vi "IMU.vi"(8 "error in (no error)":errorcluster, 10 "Acc/Gyro  address":u8, 11 "I2C Ref":T1) -> (3 "error out":errorcluster, 5 "IMU Acc":cluster{dbl, dbl, dbl}(graph), 6 "IMU Gyro":cluster{dbl, dbl, dbl}(graph))   [LabVIEW 2019]
uses:
  <vilib>/myRIO/Instrument Drivers/Onboard IO/I2C/typedefs/I2C Reference.ctl
  <vilib>/myRIO/Common/Instrument Driver Framework/Utilities/typedefs/myRIO Generic Hardware Reference.ctl
  <vilib>/myRIO/Common/Instrument Driver Framework/Utilities/typedefs/Hardware Version Enum.ctl
  <vilib>/myRIO/Common/Instrument Driver Framework/Utilities/typedefs/myRIO v1.0 Reference.ctl
  <vilib>/myRIO/Common/Instrument Driver Framework/Utilities/typedefs/Generic FPGA Reference.ctl
  <vilib>/myRIO/Common/Instrument Driver Framework/myRIO v1.0/I2C/typedefs/I2C Channels Enum.ctl
  <vilib>/myRIO/Instrument Drivers/Onboard IO/I2C/typedefs/I2C Configuration.ctl
  <vilib>/myRIO/Instrument Drivers/Onboard IO/I2C/typedefs/I2C Transfer Rate.ctl
  <vilib>/Utility/error.llb/Error Cluster From Error Code.vi
  <vilib>/myRIO/Common/Instrument Driver Framework/myRIO v1.0/I2C/vis/myRIO v1.0 Write I2C.vi
  <vilib>/myRIO/Common/Instrument Driver Framework/myRIO v1.0/I2C/vis/myRIO v1.0 Read I2C.vi
  <vilib>/myRIO/Instrument Drivers/Onboard IO/I2C/I2C.lvlib
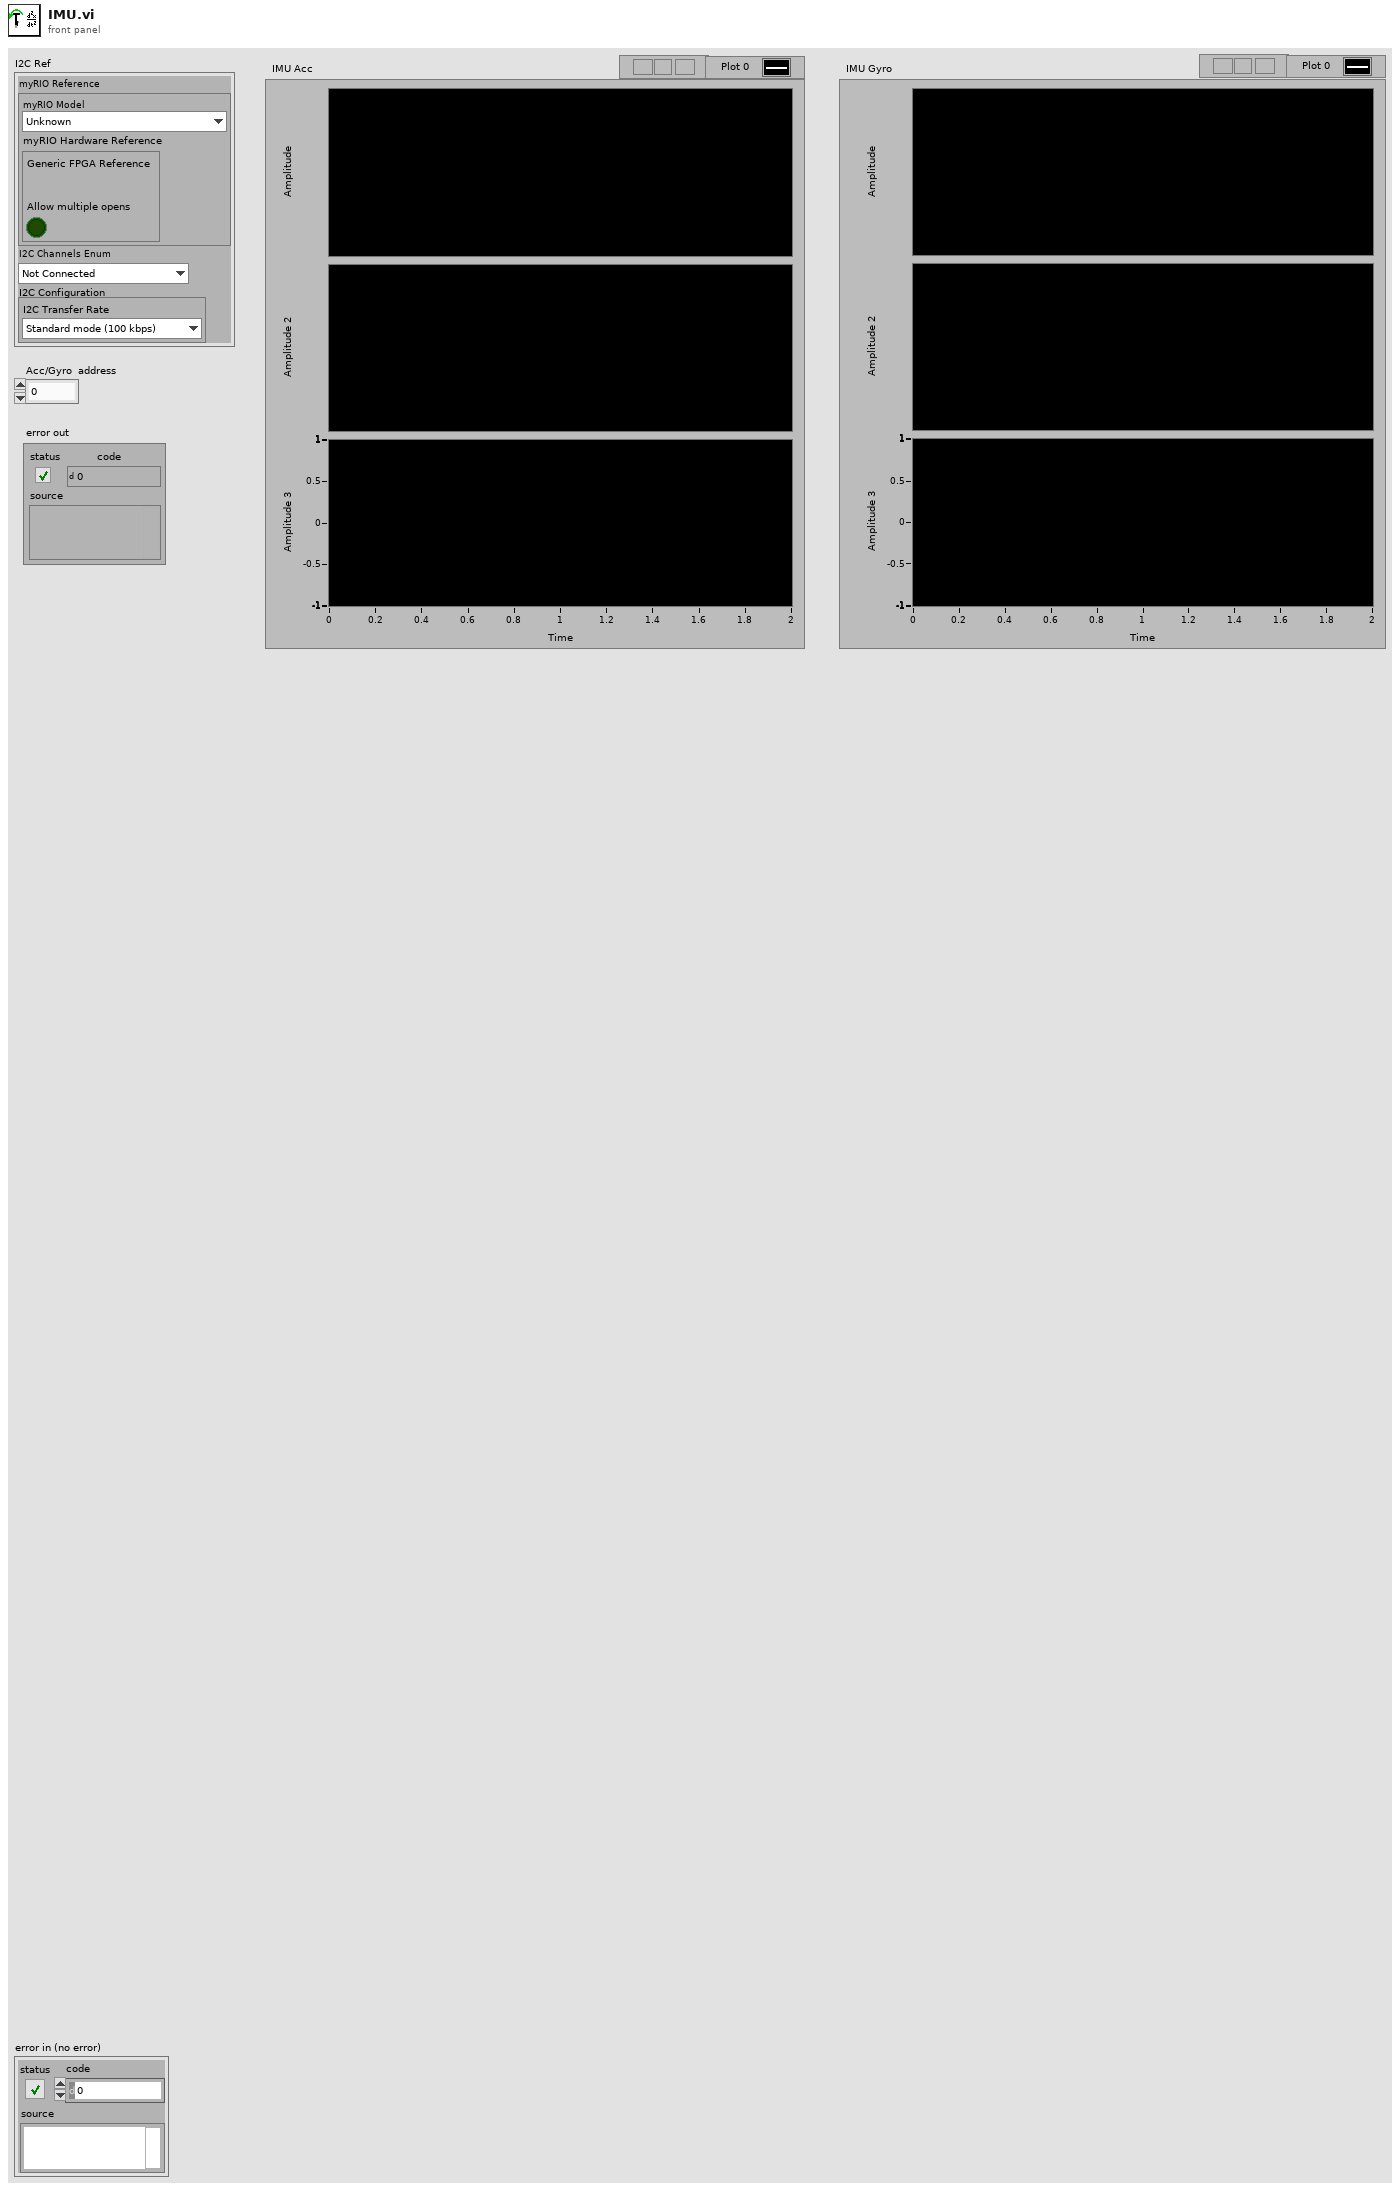
[diagram p1: front panel]
types:
  T1 = typedef "I2C.lvlib/I2C Reference.ctl" = cluster{"myRIO Reference":T2, "I2C Channels Enum":T6, "I2C Configuration":T7}
  T2 = typedef "myRIO Generic Hardware Reference.ctl" = cluster{"myRIO Model":T3, "myRIO Hardware Reference":T4}
  T3 = typedef "Hardware Version Enum.ctl" = enum16{"Unknown", "myRIO-1900", "myRIO-1950", "roboRIO", "NI ELVIS RIO CM", "ELVIS III"}
  T4 = typedef "myRIO v1.0 Reference.ctl" = cluster{"Generic FPGA Reference":T5, "Allow multiple opens":bool}
  T5 = typedef "Generic FPGA Reference.ctl" = refnum<k20>
  T6 = typedef "I2C Channels Enum.ctl" = enum16{"Not Connected", "A/I2C", "B/I2C", "I2C/I2C"}
  T7 = typedef "I2C.lvlib/I2C Configuration.ctl" = cluster{"I2C Transfer Rate":T8}
  T8 = typedef "I2C.lvlib/I2C Transfer Rate.ctl" = enum16{"Standard mode (100 kbps)", "Fast mode (400 kbps)"}
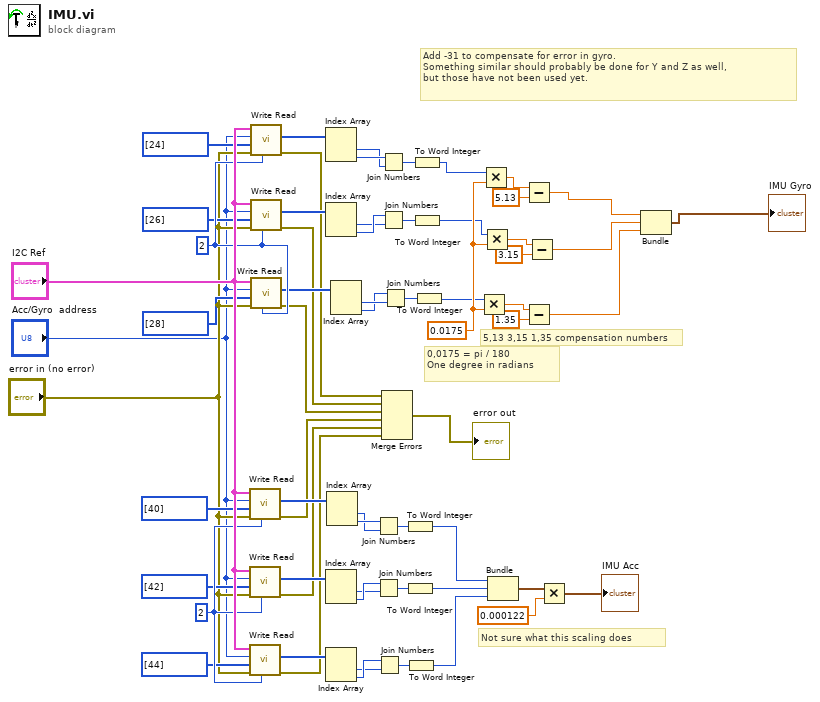
[diagram p0: block diagram]
diagram:
  w13 = 0.0175 ("y")
  w55 = u32 2 ("Byte Count")
  w41 = u32 2 ("Byte Count")
  # "5,13 3,15 1,35 compensation numbers"
  # "Add -31 to compensate for error in gyro.\nSomething similar should probably be done for Y and Z as well,\nbut those have not been used yet."
  # "0,0175 = pi / 180\nOne degree in radians"
  # "Not sure what this scaling does"
  n1 = call <vilib>:"Write Read.vi"("Byte Count"=w41, "error in (no error)"="error in (no error)", "Bytes to Write"=u8[] [40], "Slave Address (7-bit)"="Acc/Gyro  address", "I2C Ref In"="I2C Ref") -> ("error out"=w20:errorcluster, "Bytes Read"=w33:u8[])  [unwired: 3 in, 1 out]
  n2 = call <vilib>:"Write Read.vi"("Byte Count"=w41, "error in (no error)"="error in (no error)", "Bytes to Write"=u8[] [42], "Slave Address (7-bit)"="Acc/Gyro  address", "I2C Ref In"="I2C Ref") -> ("error out"=w19:errorcluster, "Bytes Read"=w31:u8[])  [unwired: 3 in, 1 out]
  n3 = call <vilib>:"Write Read.vi"("Byte Count"=w41, "error in (no error)"="error in (no error)", "Bytes to Write"=u8[] [44], "Slave Address (7-bit)"="Acc/Gyro  address", "I2C Ref In"="I2C Ref") -> ("error out"=w18:errorcluster, "Bytes Read"=w29:u8[])  [unwired: 3 in, 1 out]
  n4 = call <vilib>:"Write Read.vi"("Byte Count"=w55, "error in (no error)"="error in (no error)", "Bytes to Write"=u8[] [24], "Slave Address (7-bit)"="Acc/Gyro  address", "I2C Ref In"="I2C Ref") -> ("error out"=w23:errorcluster, "Bytes Read"=w49:u8[])  [unwired: 3 in, 1 out]
  n5 = call <vilib>:"Write Read.vi"("Byte Count"=w55, "error in (no error)"="error in (no error)", "Bytes to Write"=u8[] [26], "Slave Address (7-bit)"="Acc/Gyro  address", "I2C Ref In"="I2C Ref") -> ("error out"=w22:errorcluster, "Bytes Read"=w47:u8[])  [unwired: 3 in, 1 out]
  n6 = call <vilib>:"Write Read.vi"("Byte Count"=w55, "error in (no error)"="error in (no error)", "Bytes to Write"=u8[] [28], "Slave Address (7-bit)"="Acc/Gyro  address", "I2C Ref In"="I2C Ref") -> ("error out"=w21:errorcluster, "Bytes Read"=w45:u8[])  [unwired: 3 in, 1 out]
  n7 = Index Array "Index Array"(array=w49) -> (element #1=w51:u8, element #2=w52:u8)  [unwired: 2 in]
  n8 = Index Array "Index Array"(array=w47) -> (element #1=w53:u8, element #2=w54:u8)  [unwired: 2 in]
  n9 = Index Array "Index Array"(array=w31) -> (element #1=w37:u8, element #2=w38:u8)  [unwired: 2 in]
  n10 = Index Array "Index Array"(array=w29) -> (element #1=w39:u8, element #2=w40:u8)  [unwired: 2 in]
  n11 = Index Array "Index Array"(array=w33) -> (element #1=w35:u8, element #2=w36:u8)  [unwired: 2 in]
  n12 = Index Array "Index Array"(array=w45) -> (element #1=w16:u8, element #2=w15:u8)  [unwired: 2 in]
  n13 = Join Numbers(hi=w36, lo=w35) -> ((hi.lo)=w26:u16)
  n14 = Join Numbers(hi=w38, lo=w37) -> ((hi.lo)=w27:u16)
  n15 = Join Numbers(hi=w40, lo=w39) -> ((hi.lo)=w28:u16)
  n16 = Join Numbers(hi=w52, lo=w51) -> ((hi.lo)=w42:u16)
  n17 = Join Numbers(hi=w54, lo=w53) -> ((hi.lo)=w43:u16)
  n18 = Join Numbers(hi=w15, lo=w16) -> ((hi.lo)=w44:u16)
  n19 = Merge Errors(w23, w22, w21, w20, w19, w18) -> (→"error out":errorcluster)
  n20 = To Word Integer(number=w26) -> (16bit integer=w61:i16)
  n21 = To Word Integer(number=w27) -> (16bit integer=w60:i16)
  n22 = To Word Integer(number=w28) -> (16bit integer=w59:i16)
  n23 = To Word Integer(number=w42) -> (16bit integer=w14:i16)
  n24 = To Word Integer(number=w43) -> (16bit integer=w12:i16)
  n25 = To Word Integer(number=w44) -> (16bit integer=w11:i16)
  n26 = Multiply(x=w11, y=w13) -> (x*y=w5:dbl)
  n27 = Multiply(x=w14, y=w13) -> (x*y=w10:dbl)
  n28 = Multiply(x=w12, y=w13) -> (x*y=w4:dbl)
  n29 = Bundle "Bundle"(w61, w60, w59) -> (w57:cluster{i16, i16, i16})  [unwired: 1 in]
  n30 = Subtract(x=w10, y=5.13) -> (x-y=w9:dbl)
  n31 = Subtract(x=w5, y=1.35) -> (x-y=w2:dbl)
  n32 = Subtract(x=w4, y=3.15) -> (x-y=w3:dbl)
  n33 = Multiply(x=w57, y=0.000122) -> (x*y=→"IMU Acc":cluster{dbl, dbl, dbl})
  n34 = Bundle "Bundle"(w9, w3, w2) -> (→"IMU Gyro":cluster{dbl, dbl, dbl})  [unwired: 1 in]
